vi "Pre Launch Init.vi"(11 "Nested in":refnum<class "MainUI Panel.lvclass">) -> (0 "error out":errorcluster, 3 "Nested out":refnum<class "MainUI Panel.lvclass">)   [LabVIEW 2019, in "MainUI.lvlib" / "MainUI Panel.lvlib" / "MainUI Panel.lvclass"]
doc: "(<B>Filename</B>: Actor Framework.lvlib:Actor.lvclass:Pre Launch Init.vi)\n\nDefines behavior that occurs after the Launch Nested Actor method is invoked but before the actor's Actor Core method begins running.\n\nBy default, this method does nothing. A descendant class may override it to define behavior."
uses:
  MainUI Panel.lvclass
  MainUI Panel.lvclass/MainUI Panel.ctl
  ModuleAbstract/ModuleAbstract.lvclass
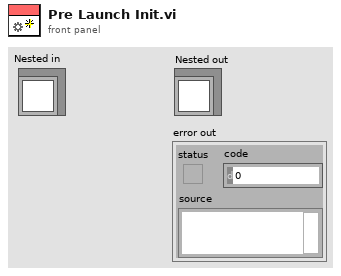
[diagram p1: front panel]
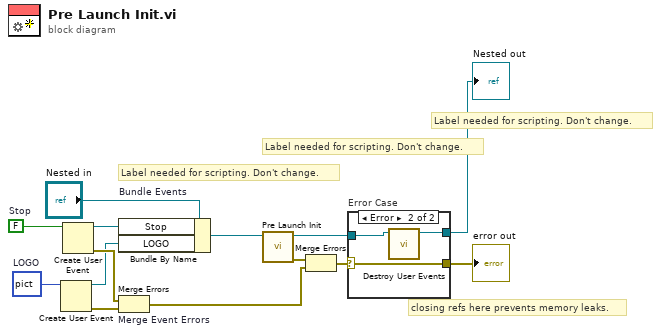
[diagram p0: block diagram]
diagram:
  w3 = picture data[5B]  # LOGO
  w13 = FALSE  # Stop
  # "Label needed for scripting. Don't change."
  # "Label needed for scripting. Don't change."
  # "Label needed for scripting. Don't change."
  # "closing refs here prevents memory leaks."
  n1 = Create User Event(user event datatype=w3) -> (user event=w2:refnum<user-event>, error out=w1:errorcluster)  [unwired: 1 in]
  n2 = Create User Event(user event datatype=w13) -> (user event=w10:refnum<user-event>, error out=w12:errorcluster)  [unwired: 1 in]
  n3 = Bundle By Name "Bundle Events"(cluster="Nested in", "Stop"=w10, "LOGO"=w2) -> (w7:refnum<class "MainUI Panel.lvclass">)
  n4 = Merge Errors "Merge Event Errors"(w12, w1) -> (w4:errorcluster)
  n5 = call-parent "Pre Launch Init.vi"("ModuleAbstract in"=w7) -> ("error out"=w6:errorcluster, "ModuleAbstract out"=w8:refnum<class "MainUI Panel.lvclass">)  [unwired: 9 in]
  n6 = Merge Errors(w6, w4) -> (w5:errorcluster)
  n7 = case "Error Case" shown="Error" w5 {
    selector: w5 -> [w15 w19]
    tunnel: w8 -> [w16 w18]
    tunnel: [w16 w17] -> w11
    tunnel: [w15 w19] -> w9
    frame No Error {
    }
    frame Error {
      n8 = call "Destroy User Events.vi"("UI Template in"=w18) -> ("UI Template out"=w17:refnum<class "MainUI Panel.lvclass">)  [unwired: 10 in]
    }
  }
  "error out" <- w9
  "Nested out" <- w11
